vi "Convert_PathWeaverJSON_To_TrajectoryFile.vi"() -> ()   [LabVIEW 2019]
uses:
  <vilib>/Rock Robotics/WPI/ThirdParty/JAS_Junk/TrajLib/TRAJ_STATE.ctl
  <vilib>/Rock Robotics/WPI/ThirdParty/JAS_Junk/TrajLib/POSE2D.ctl
  <vilib>/Rock Robotics/WPI/ThirdParty/JAS_Junk/TrajLib/TRANSLATION2D.ctl
  <vilib>/Rock Robotics/WPI/ThirdParty/JAS_Junk/TrajLib/ROTATION2D.ctl
  <vilib>/Rock Robotics/WPI/ThirdParty/JAS_Junk/TrajLib/UTIL_WAYPOINT.ctl
  <vilib>/Rock Robotics/WPI/ThirdParty/JAS_Junk/TrajLib/Trajectory_Library.lvlib
panel:
  in  "End Program":bool
  in  "Tab Control":T1(tab)
  in  "PathWeaver JSON File":path
  in  "Read JSON Fiile":bool
  out "File Read Error":errorcluster
  in  "PathWeaver Length Units":T2(radio)
  in  "WheelBase":dbl=0.6
  out "Position":cluster{dbl[], dbl[]}[](graph)
  out "Trajectory Data":cluster{dbl[], dbl[]}[](graph)
  out "Traj States\nSize":i32
  out "Trajectory States":T3[](array[typedef])
  out "File Saved\nWithout\nError":bool
  in  "Trajectory Type":enum32{"Radio Selection 1", "Radio Selection 2"}(radio)
  out "File Creation\nError":errorcluster
  in  "Trajectory File Comment":string
  in  "Trajectory File Name":path
  in  "CreateCmdList":bool
  out "Ready to\nWrite FIle":bool
  # "Convert Pathweaver JSON file to trajectory file"
  # "Instructions: \n---------------- \nThis utility reads a JSON file create from PathWeaver.  The results are plotted for review.  This file can then be written to a Trajectory Library CSV file.\n\nNotes:\n---------\n - Pathweaver sets the Y orign at the top left.  This trajectory library utilties use the bottom right.  This utility converts the Y position value to be consistent. \n   There are no consequences when the trajectory is saved as a robot relative trajectory.  For absolute trajectories, the robot position needs to\n   condier this."
  # "Meters"
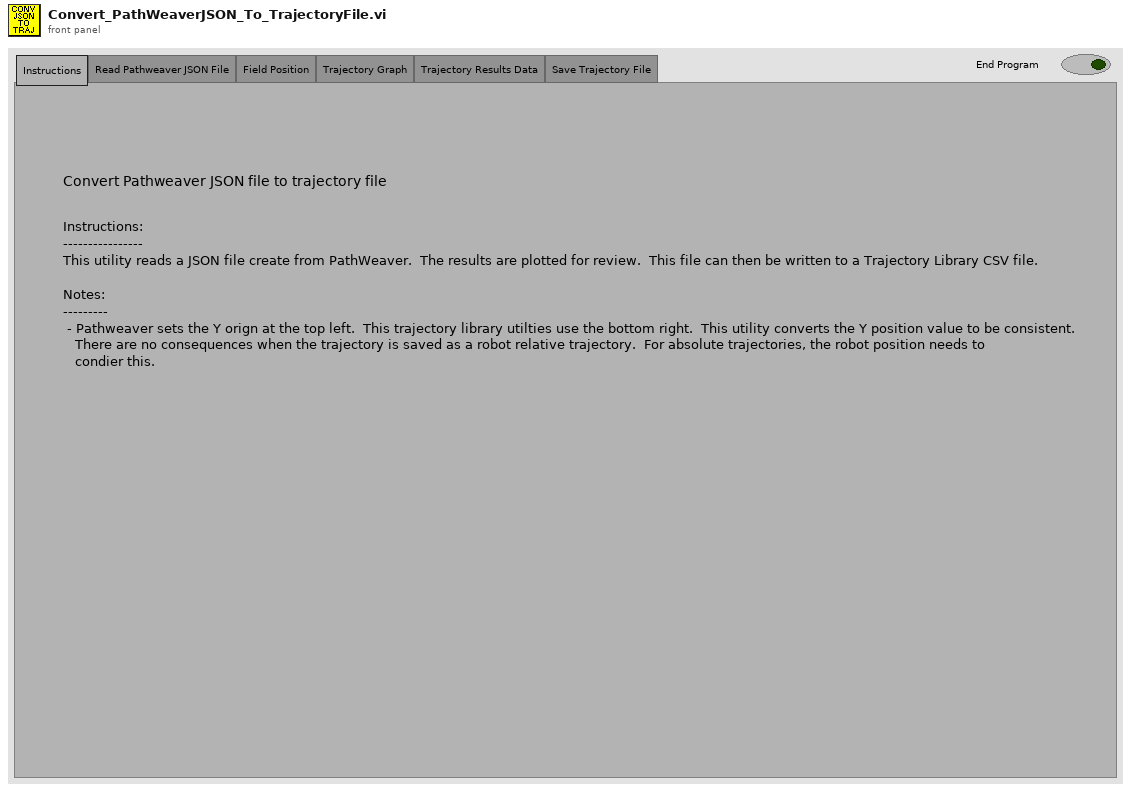
[diagram p1: front panel]
types:
  T1 = enum32{"Instructions", "Read Pathweaver JSON File", "Field Position", "Trajectory Graph", "Trajectory Results Data", "Save Trajectory File"}
  T2 = enum32{"Radio Selection 1", "Radio Selection 2", "Radio Selection 3", "Radio Selection 4", "Radio Selection 5"}
  T3 = typedef "Trajectory_Library.lvlib/TRAJ_STATE.ctl" = cluster{"TimeSeconds":dbl, "Velocity":dbl, "Acceleration":dbl, "POSE":T4, "Curvature":dbl}
  T4 = typedef "Trajectory_Library.lvlib/POSE2D.ctl" = cluster{"TRANSLATION":T5, "ROTATION":T6}
  T5 = typedef "Trajectory_Library.lvlib/TRANSLATION2D.ctl" = cluster{"X":dbl, "Y":dbl}
  T6 = typedef "Trajectory_Library.lvlib/ROTATION2D.ctl" = cluster{"VALUE":dbl, "COS":dbl, "SIN":dbl}
  T7 = typedef "Trajectory_Library.lvlib/UTIL_WAYPOINT.ctl" = cluster{"X":dbl, "Y":dbl, "ANGLE":dbl}
  T8 = typedef "Trajectory_Library.lvlib/TRAJECTORY.ctl" = cluster{"TotalTImeSecs":dbl, "States":T3[]}
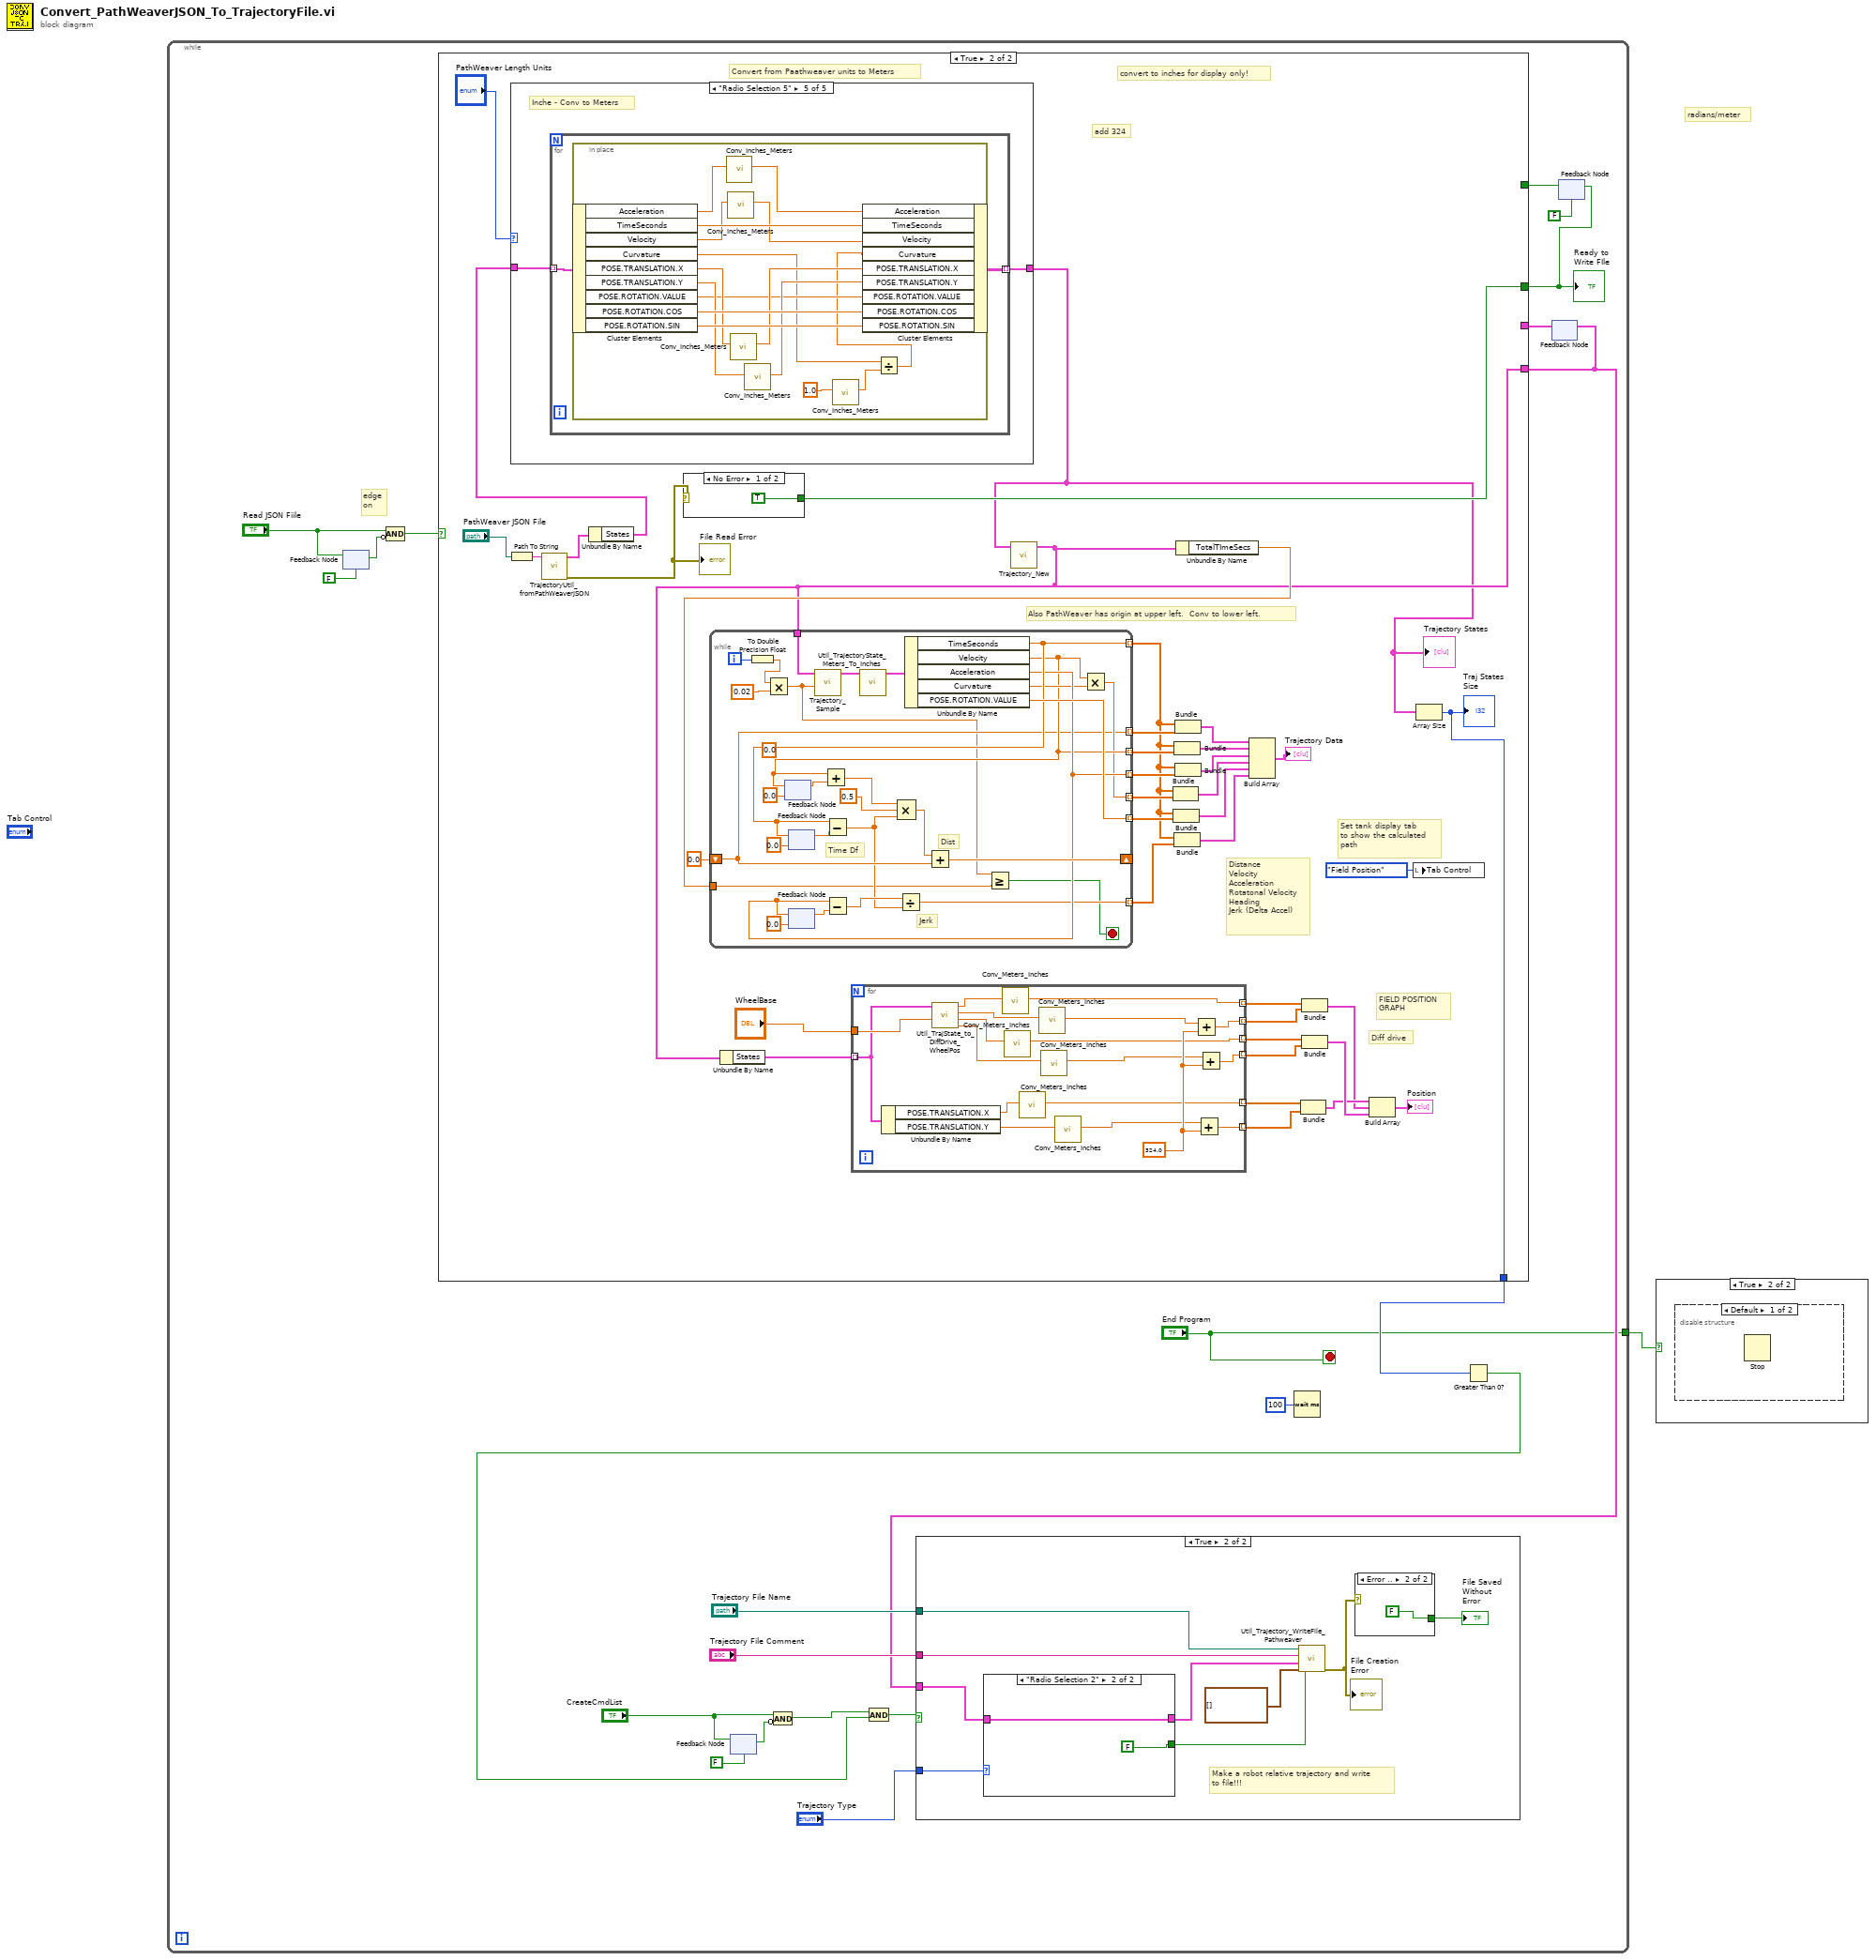
[diagram p0: block diagram]
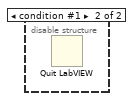
[diagram p3: hidden frame]
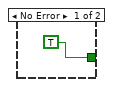
[diagram p5: hidden frame]
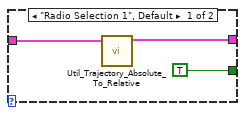
[diagram p6: hidden frame]
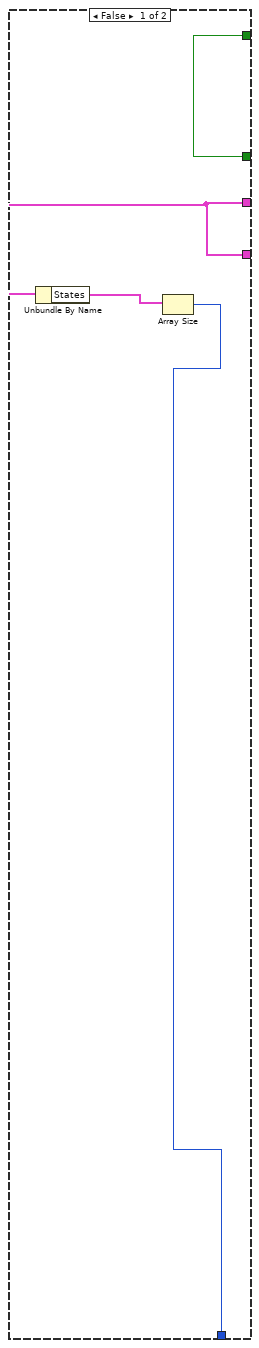
[diagram p7: hidden frame]
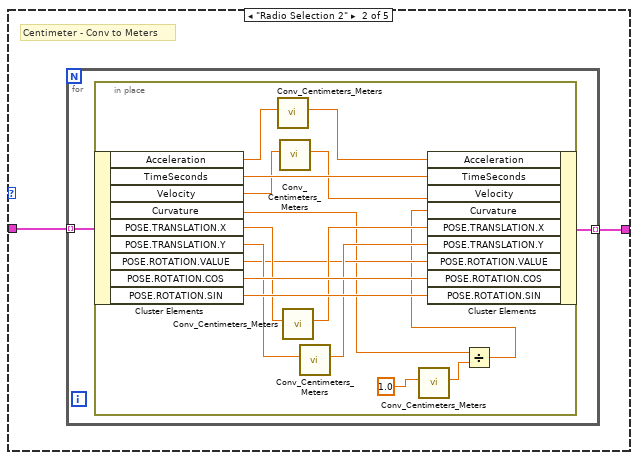
[diagram p9: hidden frame]
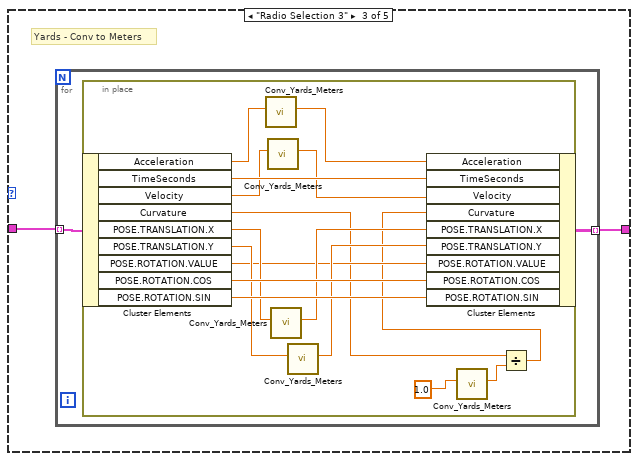
[diagram p10: hidden frame]
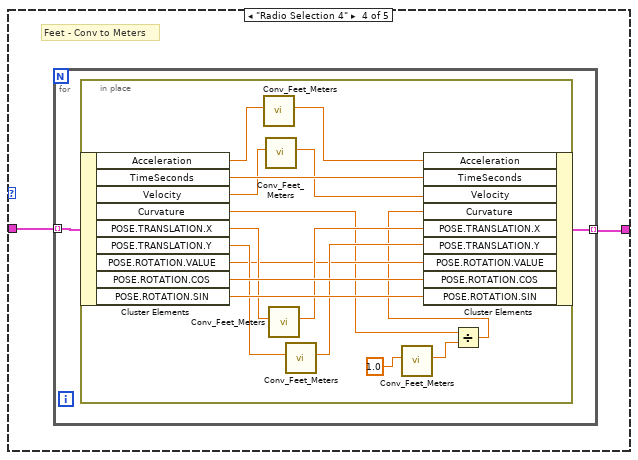
[diagram p11: hidden frame]
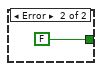
[diagram p12: hidden frame]
diagram:
  # "radians/meter"
  n1 = while {
    tunnel: ["End Program"] -> w1
    stop <- "End Program" stop-if-true
    # "edge\non"
    n2 = feedback #1(FALSE ("CreateCmdList")) -> (w11:bool)
    n3 = feedback-in #1("Read JSON Fiile") -> ()
    n4 = Compound Arithmetic op=AND("Read JSON Fiile", invert w11) -> (w9:bool)
    n5 = feedback-in #2("CreateCmdList") -> ()
    n6 = feedback #2(FALSE ("CreateCmdList")) -> (w14:bool)
    n7 = Compound Arithmetic op=AND("CreateCmdList", invert w14) -> (w13:bool)
    n8 = Wait (ms)(milliseconds to wait=u32 100) -> ()  [unwired: 1 out]
    n9 = feedback #3() -> (w21:T8)  [unwired: 1 in]
    n10 = feedback #4(FALSE) -> (w5:bool)
    n11 = case shown="True" w9 {
      tunnel: [w40 w46] -> w17
      tunnel: w21 -> [w40 _]
      tunnel: [w42 w81] -> w16
      tunnel: [w41 w77] -> w7
      tunnel: w5 -> [w41 _]
      frame False {
        n12 = Unbundle By Name(w40) -> ("States"=w39:T3[])
        n13 = Array Size(array=w39) -> (size(s)=w42:i32)
      }
      frame True {
        (unwired) 0.0
        # "add 324"
        # "Diff drive"
        # "FIELD POSITION\nGRAPH"
        # "Distance\nVelocity\nAcceleration\nRotatonal Velocity\nHeading\nJerk (Delta Accel)"
        # "Also PathWeaver has origin at upper left.  Conv to lower left."
        # "convert to inches for display only!"
        # "Convert from Paathweaver units to Meters"
        # "Set tank display tab\nto show the calculated\npath"
        n14 = Path To String(path="PathWeaver JSON File") -> (string=w80:string)
        n15 = call <vilib>:"TrajectoryUtil_fromPathWeaverJSON.vi"("FileName"=w80) -> ("error out"=w78:errorcluster, "outTRAJECTORY"=w75:T8)  [unwired: 9 in]
        "File Read Error" <- w78
        n16 = Unbundle By Name(w75) -> ("States"=w74:T3[])
        n17 = case shown="\"Radio Selection 5\"" "PathWeaver Length Units" {
          tunnel: w74 -> [w129 w130 w151 w171 w191]
          tunnel: [w129 w131 w150 w170 w190] -> w43
          frame "Radio Selection 1" {
            # "Meters - do nothing"
          }
          frame "Radio Selection 2" {
            # "Centimeter - Conv to Meters"
            n18 = for {
              tunnel: w130 -> [w133] mode=indexing
              tunnel: [w132] -> w131 mode=indexing
              n19 = in-place {
                n20 = in-place-cluster #5(w133) -> ("Acceleration"=w141:dbl, "TimeSeconds"=w149:dbl, "Velocity"=w143:dbl, "Curvature"=w134:dbl, "POSE.TRANSLATION.X"=w145:dbl, "POSE.TRANSLATION.Y"=w146:dbl, "POSE.ROTATION.VALUE"=w138:dbl, "POSE.ROTATION.COS"=w148:dbl, "POSE.ROTATION.SIN"=w147:dbl)
                n21 = call <vilib>:"Conv_Centimeters_Meters.vi"("Centimeter"=w141) -> ("Meters"=w140:dbl)  [unwired: 10 in]
                n22 = call <vilib>:"Conv_Centimeters_Meters.vi"("Centimeter"=w143) -> ("Meters"=w142:dbl)  [unwired: 10 in]
                n23 = call <vilib>:"Conv_Centimeters_Meters.vi"("Centimeter"=w145) -> ("Meters"=w144:dbl)  [unwired: 10 in]
                n24 = call <vilib>:"Conv_Centimeters_Meters.vi"("Centimeter"=w146) -> ("Meters"=w139:dbl)  [unwired: 10 in]
                n25 = call <vilib>:"Conv_Centimeters_Meters.vi"("Centimeter"=1.0) -> ("Meters"=w135:dbl)  [unwired: 10 in]
                n26 = Divide(x=w134, y=w135) -> (x/y=w137:dbl)
                n27 = in-place-cluster #5("Acceleration"=w140, "TimeSeconds"=w149, "Velocity"=w142, "Curvature"=w137, "POSE.TRANSLATION.X"=w144, "POSE.TRANSLATION.Y"=w139, "POSE.ROTATION.VALUE"=w138, "POSE.ROTATION.COS"=w148, "POSE.ROTATION.SIN"=w147) -> (w132:T3)
              }
            }
          }
          frame "Radio Selection 3" {
            # "Yards - Conv to Meters"
            n28 = for {
              tunnel: w151 -> [w153] mode=indexing
              tunnel: [w152] -> w150 mode=indexing
              n29 = in-place {
                n30 = in-place-cluster #6(w153) -> ("Acceleration"=w161:dbl, "TimeSeconds"=w169:dbl, "Velocity"=w163:dbl, "Curvature"=w157:dbl, "POSE.TRANSLATION.X"=w165:dbl, "POSE.TRANSLATION.Y"=w166:dbl, "POSE.ROTATION.VALUE"=w158:dbl, "POSE.ROTATION.COS"=w168:dbl, "POSE.ROTATION.SIN"=w167:dbl)
                n31 = call <vilib>:"Conv_Yards_Meters.vi"("Yards"=w161) -> ("Meters"=w160:dbl)  [unwired: 10 in]
                n32 = call <vilib>:"Conv_Yards_Meters.vi"("Yards"=w163) -> ("Meters"=w162:dbl)  [unwired: 10 in]
                n33 = call <vilib>:"Conv_Yards_Meters.vi"("Yards"=w165) -> ("Meters"=w164:dbl)  [unwired: 10 in]
                n34 = call <vilib>:"Conv_Yards_Meters.vi"("Yards"=w166) -> ("Meters"=w159:dbl)  [unwired: 10 in]
                n35 = call <vilib>:"Conv_Yards_Meters.vi"("Yards"=1.0 ("Centimeter")) -> ("Meters"=w155:dbl)  [unwired: 10 in]
                n36 = Divide(x=w157, y=w155) -> (x/y=w156:dbl)
                n37 = in-place-cluster #6("Acceleration"=w160, "TimeSeconds"=w169, "Velocity"=w162, "Curvature"=w156, "POSE.TRANSLATION.X"=w164, "POSE.TRANSLATION.Y"=w159, "POSE.ROTATION.VALUE"=w158, "POSE.ROTATION.COS"=w168, "POSE.ROTATION.SIN"=w167) -> (w152:T3)
              }
            }
          }
          frame "Radio Selection 4" {
            # "Feet - Conv to Meters"
            n38 = for {
              tunnel: w171 -> [w173] mode=indexing
              tunnel: [w172] -> w170 mode=indexing
              n39 = in-place {
                n40 = in-place-cluster #7(w173) -> ("Acceleration"=w181:dbl, "TimeSeconds"=w189:dbl, "Velocity"=w183:dbl, "Curvature"=w175:dbl, "POSE.TRANSLATION.X"=w185:dbl, "POSE.TRANSLATION.Y"=w186:dbl, "POSE.ROTATION.VALUE"=w178:dbl, "POSE.ROTATION.COS"=w188:dbl, "POSE.ROTATION.SIN"=w187:dbl)
                n41 = call <vilib>:"Conv_Feet_Meters.vi"("Feet"=w181) -> ("Meters"=w180:dbl)  [unwired: 10 in]
                n42 = call <vilib>:"Conv_Feet_Meters.vi"("Feet"=w183) -> ("Meters"=w182:dbl)  [unwired: 10 in]
                n43 = call <vilib>:"Conv_Feet_Meters.vi"("Feet"=w185) -> ("Meters"=w184:dbl)  [unwired: 10 in]
                n44 = call <vilib>:"Conv_Feet_Meters.vi"("Feet"=w186) -> ("Meters"=w179:dbl)  [unwired: 10 in]
                n45 = call <vilib>:"Conv_Feet_Meters.vi"("Feet"=1.0 ("Centimeter")) -> ("Meters"=w176:dbl)  [unwired: 10 in]
                n46 = Divide(x=w175, y=w176) -> (x/y=w174:dbl)
                n47 = in-place-cluster #7("Acceleration"=w180, "TimeSeconds"=w189, "Velocity"=w182, "Curvature"=w174, "POSE.TRANSLATION.X"=w184, "POSE.TRANSLATION.Y"=w179, "POSE.ROTATION.VALUE"=w178, "POSE.ROTATION.COS"=w188, "POSE.ROTATION.SIN"=w187) -> (w172:T3)
              }
            }
          }
          frame "Radio Selection 5" {
            # "Inche - Conv to Meters"
            n48 = for {
              tunnel: w191 -> [w193] mode=indexing
              tunnel: [w192] -> w190 mode=indexing
              n49 = in-place {
                n50 = in-place-cluster #8(w193) -> ("Acceleration"=w201:dbl, "TimeSeconds"=w209:dbl, "Velocity"=w203:dbl, "Curvature"=w195:dbl, "POSE.TRANSLATION.X"=w205:dbl, "POSE.TRANSLATION.Y"=w206:dbl, "POSE.ROTATION.VALUE"=w198:dbl, "POSE.ROTATION.COS"=w208:dbl, "POSE.ROTATION.SIN"=w207:dbl)
                n51 = call <vilib>:"Conv_Inches_Meters.vi"("INCH"=w201) -> ("Meters"=w200:dbl)  [unwired: 10 in]
                n52 = call <vilib>:"Conv_Inches_Meters.vi"("INCH"=w203) -> ("Meters"=w202:dbl)  [unwired: 10 in]
                n53 = call <vilib>:"Conv_Inches_Meters.vi"("INCH"=w205) -> ("Meters"=w204:dbl)  [unwired: 10 in]
                n54 = call <vilib>:"Conv_Inches_Meters.vi"("INCH"=w206) -> ("Meters"=w199:dbl)  [unwired: 10 in]
                n55 = call <vilib>:"Conv_Inches_Meters.vi"("INCH"=1.0 ("Centimeter")) -> ("Meters"=w196:dbl)  [unwired: 10 in]
                n56 = Divide(x=w195, y=w196) -> (x/y=w194:dbl)
                n57 = in-place-cluster #8("Acceleration"=w200, "TimeSeconds"=w209, "Velocity"=w202, "Curvature"=w194, "POSE.TRANSLATION.X"=w204, "POSE.TRANSLATION.Y"=w199, "POSE.ROTATION.VALUE"=w198, "POSE.ROTATION.COS"=w208, "POSE.ROTATION.SIN"=w207) -> (w192:T3)
              }
            }
          }
        }
        "Trajectory States" <- w43
        n58 = case shown="No Error" w78 {
          tunnel: [TRUE FALSE] -> w77
          frame No Error {
          }
          frame Error {
          }
        }
        n59 = call <vilib>:"Trajectory_New.vi"("TRAJ_STATES"=w43) -> ("TRAJECTORY"=w46:T8)  [unwired: 10 in]
        n60 = Unbundle By Name(w46) -> ("States"=w45:T3[])
        n61 = for {
          tunnel: w45 -> [w94] mode=indexing
          tunnel: "WheelBase" -> [w99]
          tunnel: [w88] -> w55 mode=indexing
          tunnel: [w90] -> w54 mode=indexing
          tunnel: [w86] -> w53 mode=indexing
          tunnel: [w89] -> w52 mode=indexing
          tunnel: [w83] -> w48 mode=indexing
          tunnel: [w84] -> w47 mode=indexing
          w91 = 324.0 ("y")
          n62 = Unbundle By Name(w94) -> ("POSE.TRANSLATION.X"=w93:dbl, "POSE.TRANSLATION.Y"=w92:dbl)
          n63 = call <vilib>:"Util_TrajState_to_DiffDrive_WheelPos.vi"("Wheelbase"=w99, "TRAJ_STATE"=w94) -> ("Right Y"=w95:dbl, "Right X"=w96:dbl, "Left Y"=w97:dbl, "Left X"=w98:dbl)  [unwired: 6 in]
          n64 = call <vilib>:"Conv_Meters_Inches.vi"("Meters"=w98) -> ("Inches"=w88:dbl)  [unwired: 10 in]
          n65 = call <vilib>:"Conv_Meters_Inches.vi"("Meters"=w96) -> ("Inches"=w86:dbl)  [unwired: 10 in]
          n66 = call <vilib>:"Conv_Meters_Inches.vi"("Meters"=w93) -> ("Inches"=w84:dbl)  [unwired: 10 in]
          n67 = call <vilib>:"Conv_Meters_Inches.vi"("Meters"=w97) -> ("Inches"=w87:dbl)  [unwired: 10 in]
          n68 = call <vilib>:"Conv_Meters_Inches.vi"("Meters"=w95) -> ("Inches"=w85:dbl)  [unwired: 10 in]
          n69 = call <vilib>:"Conv_Meters_Inches.vi"("Meters"=w92) -> ("Inches"=w82:dbl)  [unwired: 10 in]
          n70 = Add(x=w87, y=w91) -> (x+y=w90:dbl)
          n71 = Add(x=w82, y=w91) -> (x+y=w83:dbl)
          n72 = Add(x=w85, y=w91) -> (x+y=w89:dbl)
        }
        n73 = Unbundle By Name(w46) -> ("TotalTImeSecs"=w58:dbl)
        n74 = while {
          tunnel: [w121] -> w60 mode=indexing
          tunnel: [w112] -> w70 mode=indexing
          tunnel: [w114] -> w69 mode=indexing
          tunnel: [w118] -> w68 mode=indexing
          tunnel: [w113] -> w67 mode=indexing
          tunnel: [w128] -> w66 mode=indexing
          shift-right: [w122] -> _
          shift-left: 0.0 -> [w112]
          tunnel: [w116] -> w59 mode=indexing
          tunnel: w58 -> [w108]
          tunnel: w46 -> [w106]
          i -> [w105]
          stop <- w107 stop-if-true
          # "Time Df"
          # "Jerk"
          # "Dist"
          n75 = To Double Precision Float(number=w105) -> (double precision float=w104:dbl)
          n76 = Multiply(x=w104, y=0.02) -> (x*y=w102:dbl)
          n77 = feedback #9(0.0 ("TimeSeconds")) -> (w124:dbl)
          n78 = feedback #10(0.0 ("TimeSeconds")) -> (w126:dbl)
          n79 = feedback #11(0.0 ("TimeSeconds")) -> (w119:dbl)
          n80 = call <vilib>:"Trajectory_Sample.vi"("Time"=w102, "InputTRAJECTORY"=w106) -> ("OutputTRAJ_STATE"=w100:T3)  [unwired: 9 in]
          n81 = call <vilib>:"Util_TrajectoryState_Meters_To_Inches.vi"("absTRAJECTORY"=w100) -> ("outputRelativeTRAJECTORY"=w101:T3)  [unwired: 10 in]
          n82 = Unbundle By Name(w101) -> ("TimeSeconds"=w121:dbl, "Velocity"=w114:dbl, "Acceleration"=w118:dbl, "Curvature"=w115:dbl, "POSE.ROTATION.VALUE"=w128:dbl)
          n83 = feedback-in #9(w114) -> ()
          n84 = feedback-in #10(w121) -> ()
          n85 = feedback-in #11(w118) -> ()
          n86 = Add(x=w114, y=w124) -> (x+y=w123:dbl)
          n87 = Subtract(x=w121, y=w126) -> (x-y=w109:dbl)
          n88 = Subtract(x=w118, y=w119) -> (x-y=w117:dbl)
          n89 = Compound Arithmetic op=MULTIPLY(w123, 0.5 ("value"), w109) -> (w111:dbl)
          n90 = Divide(x=w117, y=w109) -> (x/y=w116:dbl)
          n91 = Add(x=w111, y=w112) -> (x+y=w122:dbl)
          n92 = Greater Or Equal?(x=w102, y=w108) -> (x >= y?=w107:bool)
          n93 = Multiply(x=w114, y=w115) -> (x*y=w113:dbl)
        }
        n94 = Bundle(w60, w67) -> (w65:cluster{dbl[], dbl[]})  [unwired: 1 in]
        n95 = Bundle(w60, w66) -> (w64:cluster{dbl[], dbl[]})  [unwired: 1 in]
        n96 = Bundle(w60, w69) -> (w72:cluster{dbl[], dbl[]})  [unwired: 1 in]
        n97 = Bundle(w60, w59) -> (w61:cluster{dbl[], dbl[]})  [unwired: 1 in]
        n98 = Bundle(w60, w70) -> (w73:cluster{dbl[], dbl[]})  [unwired: 1 in]
        n99 = Bundle(w60, w68) -> (w71:cluster{dbl[], dbl[]})  [unwired: 1 in]
        n100 = Build Array(w73, w72, w71, w65, w64, w61) -> (→"Trajectory Data":cluster{dbl[], dbl[]}[])
        n101 = Bundle(w47, w48) -> (w50:cluster{dbl[], dbl[]})  [unwired: 1 in]
        n102 = Bundle(w55, w54) -> (w49:cluster{dbl[], dbl[]})  [unwired: 1 in]
        n103 = Bundle(w53, w52) -> (w51:cluster{dbl[], dbl[]})  [unwired: 1 in]
        n104 = Build Array(w50, w49, w51) -> (→"Position":cluster{dbl[], dbl[]}[])
        n105 = local write "Tab Control"(T1."Field Position" ("Tab Control")) -> ()
        n106 = Array Size(array=w43) -> (size(s)=w81:i32)
        "Traj States\nSize" <- w81
      }
    }
    "Ready to\nWrite FIle" <- w7
    n107 = Greater Than 0?(x=w16) -> (x > 0?=w4:bool)
    n108 = And(x=w13, y=w4) -> (x .and. y?=w18:bool)
    n109 = case shown="True" w18 {
      tunnel: "Trajectory File Name" -> [_ w31]
      tunnel: "Trajectory File Comment" -> [_ w30]
      tunnel: w17 -> [_ w27]
      tunnel: "Trajectory Type" -> [_ w28]
      frame False {
      }
      frame True {
        # "Make a robot relative trajectory and write\nto file!!!"
        n110 = case shown="\"Radio Selection 2\"" w28 {
          tunnel: w27 -> [w36 w38]
          tunnel: [w35 w38] -> w26
          tunnel: [TRUE FALSE] -> w23
          frame "Radio Selection 1", Default {
            n111 = call <vilib>:"Util_Trajectory_Absolute_To_Relative.vi"("absTRAJECTORY"=w36) -> ("outputRelativeTRAJECTORY"=w35:T8)  [unwired: 10 in]
          }
          frame "Radio Selection 2" {
          }
        }
        n112 = call <vilib>:"Util_Trajectory_WriteFile_Pathweaver.vi"("Trajectory Is Relative"=w23, "UtilityWayPoints"=T7[] [], "TRAJECTORY"=w26, "Comment"=w30, "Trajectory File Name"=w31) -> ("error out"=w25:errorcluster)  [unwired: 6 in]
        "File Creation\nError" <- w25
        n113 = case shown="Error .." w25 {
          tunnel: [TRUE ("File Saved\nWithout\nError") FALSE ("File Saved\nWithout\nError")] -> w24
          frame No Error {
          }
          frame Error {
          }
        }
        "File Saved\nWithout\nError" <- w24
      }
    }
    n114 = feedback-in #3(w17) -> ()
    n115 = feedback-in #4(w7) -> ()
  }
  n116 = case shown="True" w1 {
    frame False {
    }
    frame True {
      n117 = disable-structure shown="Default" {
        frame condition #0 (active) {
          n118 = Stop() -> ()  [unwired: 1 in]
        }
        frame condition #1 {
          n119 = Quit LabVIEW() -> ()  [unwired: 1 in]
        }
      }
    }
  }
